vi "BRig_Host_dataRunState_entryAdd_trig.vi"(7 "input_idx":i32[](array[numeric]), 8 "input_trig_l2":u16, 9 "input_trig_l1":u16, 10 "input_nTrial":u16, 11 "input_dataPlot":u16[][](array[numeric])) -> (3 "output_dataPlot":u16[][](array[numeric]), 5 "output_idx":i32[](array[numeric]))   [LabVIEW 2014]
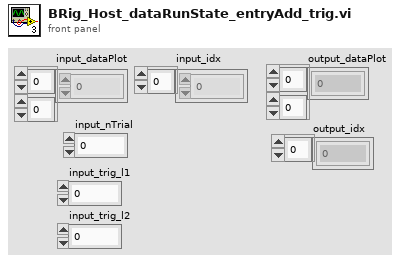
[diagram p1: front panel]
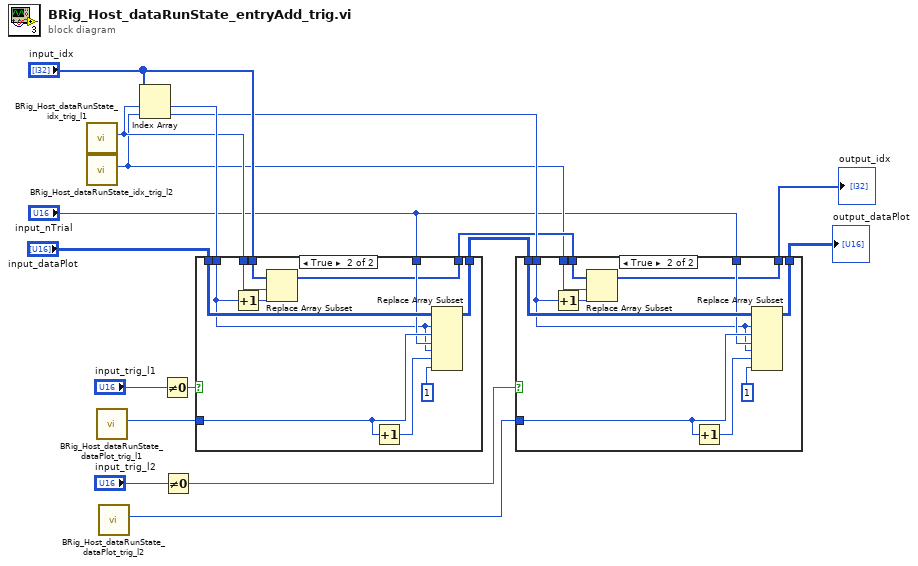
[diagram p0: block diagram]
diagram:
  n1 = call "BRig_Host_dataRunState_idx_trig_l1.vi"() -> ("output_idx_trig_l1"=w11:i32)  [unwired: 11 in]
  n2 = call "BRig_Host_dataRunState_idx_trig_l2.vi"() -> ("output_idx_trig_l2"=w6:i32)  [unwired: 11 in]
  n3 = call "BRig_Host_dataRunState_dataPlot_trig_l1.vi"() -> ("output_idx_dataPlot_trig_l1"=w14:i32)  [unwired: 11 in]
  n4 = call "BRig_Host_dataRunState_dataPlot_trig_l2.vi"() -> ("output_idx_dataPlot_trig_l2"=w4:i32)  [unwired: 11 in]
  n5 = Index Array(array="input_idx", index #1=w11, index #2=w6) -> (element #1=w12:i32, element #2=w8:i32)
  n6 = Not Equal To 0?(x="input_trig_l1") -> (x != 0?=w16:bool)
  n7 = Not Equal To 0?(x="input_trig_l2") -> (x != 0?=w5:bool)
  n8 = case shown="True" w16 {
    tunnel: w12 -> [_ w20]
    tunnel: "input_dataPlot" -> [w19 w30]
    tunnel: w14 -> [_ w29]
    tunnel: "input_nTrial" -> [_ w27]
    tunnel: [w19 w25] -> w9
    tunnel: w11 -> [_ w24]
    tunnel: "input_idx" -> [w18 w23]
    tunnel: [w18 w21] -> w7
    frame False {
    }
    frame True {
      n9 = Increment(x=w20) -> (x+1=w22:i32)
      n10 = Replace Array Subset(array=w23, new element=w22, index=w24) -> (w21:i32[])
      n11 = Increment(x=w29) -> (x+1=w28:i32)
      n12 = Replace Array Subset(array=w30, new element #1=w27, index (row) #1=w20, index (col) #1=w29, new element #2=u16 1 ("new element/subarray"), index (row) #2=w20, index (col) #2=w28) -> (w25:u16[][])
    }
  }
  n13 = case shown="True" w5 {
    tunnel: w8 -> [_ w33]
    tunnel: w9 -> [w32 w43]
    tunnel: w4 -> [_ w42]
    tunnel: "input_nTrial" -> [_ w40]
    tunnel: [w32 w38] -> w2
    tunnel: w6 -> [_ w37]
    tunnel: w7 -> [w31 w36]
    tunnel: [w31 w34] -> w1
    frame False {
    }
    frame True {
      n14 = Increment(x=w33) -> (x+1=w35:i32)
      n15 = Replace Array Subset(array=w36, new element=w35, index=w37) -> (w34:i32[])
      n16 = Increment(x=w42) -> (x+1=w41:i32)
      n17 = Replace Array Subset(array=w43, new element #1=w40, index (row) #1=w33, index (col) #1=w42, new element #2=u16 1 ("new element/subarray"), index (row) #2=w33, index (col) #2=w41) -> (w38:u16[][])
    }
  }
  "output_dataPlot" <- w2
  "output_idx" <- w1
